vi "User Access Level FGV Unit Test-new.vi"() -> ()   [LabVIEW 2013]
uses:
  User Level FGV/User Access Level Method.ctl
panel:
  in  "访问安全区域":bool
  out "错误输出":cluster{"状态":bool, "代码":i32, "源":string}
  in  "错误输入":cluster{"状态":bool, "代码":i32, "源":string}
  in  "当前用户":string
  in  "设置用户访问级别":bool
  in  "停止":bool
  # "1.  为当前用户设置访问级别。"
  # "2.  通过验证对话框消息，测试访问级别。"
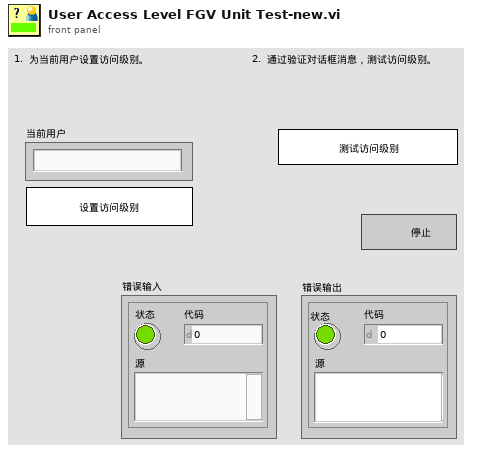
[diagram p1: front panel]
types:
  T1 = typedef "User Access Level Method.ctl" = enum16{"读取用户访问级别文件", "设置当前访问级别", "获取当前访问级别"}
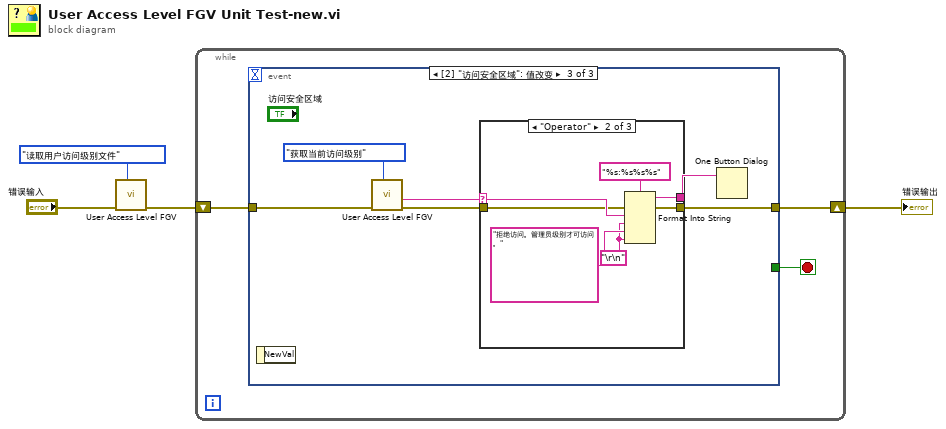
[diagram p0: block diagram]
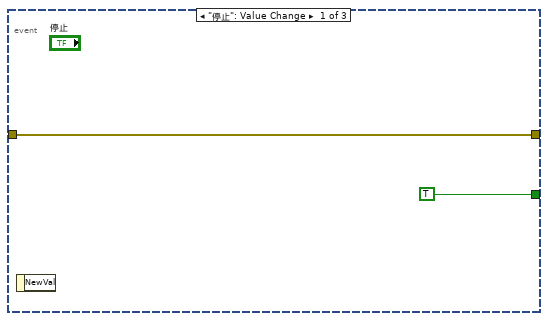
[diagram p2: hidden frame]
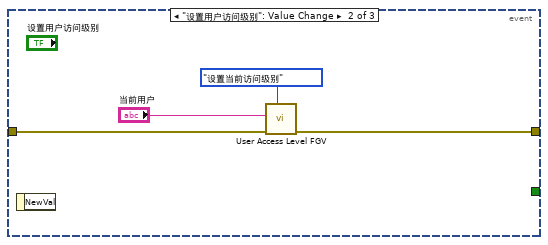
[diagram p3: hidden frame]
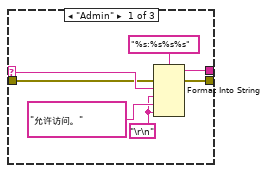
[diagram p4: hidden frame]
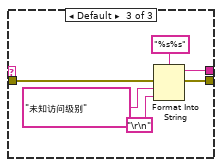
[diagram p5: hidden frame]
diagram:
  n1 = call "User Access Level FGV.vi"("用户等级命令"=User_Access_Level_Method."读取用户访问级别文件", "错误输入"="错误输入") -> ("错误输出"=w4:cluster{"状态":bool, "代码":i32, "源":string})  [unwired: 8 in, 1 out]
  n2 = while {
    shift-right: [w5] -> w1
    shift-left: w4 -> [w6]
    stop <- w7 stop-if-true
    n3 = event shown="[2] \"访问安全区域\": 值改变" {
      selector: _ -> [_ _ _]
      dyn-events: _ -> [_ _ _]
      timeout: _ -> [_ _ _]
      tunnel: [TRUE ("停止") _ _] -> w7
      tunnel: w6 -> [w8 w12 w18]
      tunnel: [w8 w10 w17] -> w5
      event "停止": Value Change {
        n4 = event-data ("事件数据节点")() -> ()  [unwired: 1 in, 1 out]
      }
      event "设置用户访问级别": Value Change {
        n5 = event-data ("事件数据节点")() -> ()  [unwired: 1 in, 1 out]
        n6 = call "User Access Level FGV.vi"("用户等级命令"=User_Access_Level_Method."设置当前访问级别", "错误输入"=w12, "用户名"="当前用户") -> ("错误输出"=w10:cluster{"状态":bool, "代码":i32, "源":string})  [unwired: 7 in, 1 out]
      }
      event "访问安全区域": Value Change {
        n7 = event-data ("事件数据节点")() -> ()  [unwired: 1 in, 1 out]
        n8 = call "User Access Level FGV.vi"("用户等级命令"=User_Access_Level_Method."获取当前访问级别", "错误输入"=w18) -> ("错误输出"=w16:cluster{"状态":bool, "代码":i32, "源":string}, "用户级别"=w15:string)  [unwired: 8 in]
        n9 = case shown="\"Operator\"" w15 {
          selector: w15 -> [w26 w33 _]
          tunnel: [w24 w31 w38] -> w17
          tunnel: w16 -> [w25 w32 w39]
          tunnel: [w20 w27 w36] -> w14
          frame "Admin" {
            w22 = "\r\n" ("行结束常量")
            n10 = Format Into String ("格式化写入字符串")(format string="%s:%s%s%s" ("格式字符串"), error in=w25, w26, w22, "允许访问。" ("消息"), w22) -> (resulting string=w20:string, error out=w24:errorcluster)  [unwired: 1 in]
          }
          frame "Operator" {
            w29 = "\r\n" ("行结束常量")
            n11 = Format Into String ("格式化写入字符串")(format string="%s:%s%s%s" ("格式字符串"), error in=w32, w33, w29, "拒绝访问。管理员级别才可访问。" ("消息"), w29) -> (resulting string=w27:string, error out=w31:errorcluster)  [unwired: 1 in]
          }
          frame Default {
            n12 = Format Into String ("格式化写入字符串")(format string="%s%s" ("格式字符串"), error in=w39, "未知访问级别" ("消息"), "\r\n" ("行结束常量")) -> (resulting string=w36:string, error out=w38:errorcluster)  [unwired: 1 in]
          }
        }
        n13 = One Button Dialog ("单按钮对话框")(message=w14) -> ()  [unwired: 1 in, 1 out]
      }
    }
  }
  "错误输出" <- w1
